vi "Get Temperature.vi"(4 "Channel":i32, 8 "error in (no error)":errorcluster, 11 "instrument.PPMS2 in":refnum<class "instrument.PPMS2.lvclass">) -> (0 "error out":errorcluster, 1 "Status":variant, 2 "Temperature (K)":dbl, 3 "instrument.PPMS2 out":refnum<class "instrument.PPMS2.lvclass">)   [LabVIEW 2016, in "instrument.PPMS2.lvclass"]
uses:
  <userlib>/LevyLab/PPMS2 Instrument/instrument.PPMS2/instrument.PPMS2.lvclass
  <userlib>/LevyLab/PPMS2 Instrument/instrument.PPMS2/Typedefs/Temperature Status--PPMS2--cluster.ctl
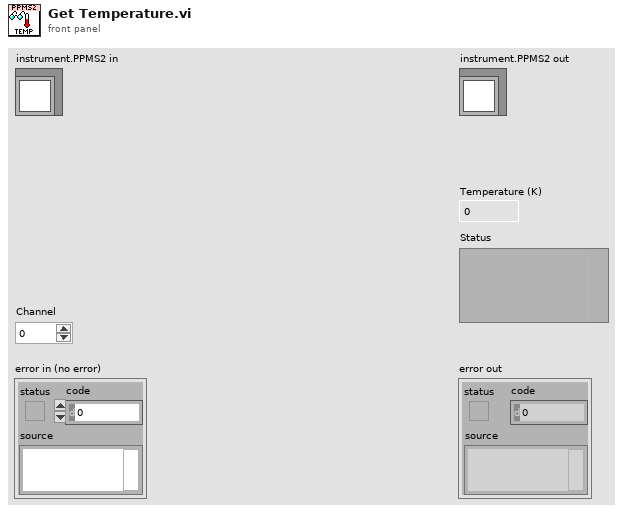
[diagram p1: front panel]
types:
  T1 = typedef "instrument.PPMS2.lvclass/Temperature Status--PPMS2--cluster.ctl" = cluster{"Temperature (K)":dbl, "Temperature Status":i32}
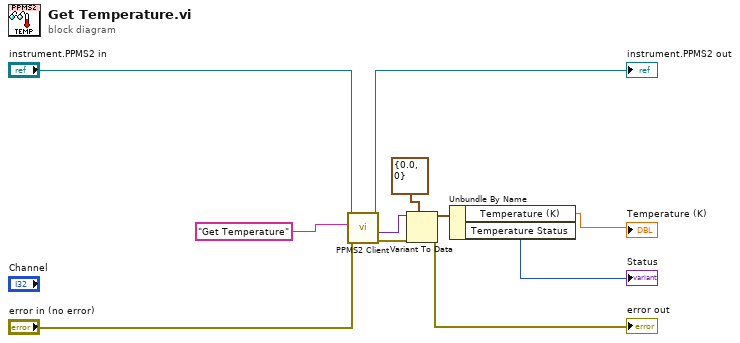
[diagram p0: block diagram]
diagram:
  n1 = call <userlib>:"PPMS2 Client.vi"("error in (no error)"="error in (no error)", "Command"="Get Temperature", "instrument.PPMS2 in"="instrument.PPMS2 in") -> ("error out"=w2:errorcluster, "Data out"=w1:variant, "instrument.PPMS2 out"=→"instrument.PPMS2 out":refnum<class "instrument.PPMS2.lvclass">)  [unwired: 5 in, 1 out]
  n2 = Variant To Data(error in=w2, type=T1 {"Temperature (K)"=0.0, "Temperature Status"=0} ("Temperature Status"), Variant=w1) -> (data=w4:T1, error out=→"error out":errorcluster)
  n3 = Unbundle By Name(w4) -> ("Temperature (K)"=→"Temperature (K)":dbl, "Temperature Status"=→"Status":i32)
